vi "数据查询_报警信息.vi"() -> ()   [LabVIEW 2016, in "数据查询.lvlib"]
uses:
  <vilib>/Utility/miscctls.llb/LVPointTypeDef.ctl
  <vilib>/Utility/miscctls.llb/LVRowAndColumnUnsignedTypeDef.ctl
  <userlib>/_OpenG.lib/array/array.llb/Remove Duplicates from 1D Array (String)__ogtk.vi
  <userlib>/_OpenG.lib/array/array.llb/Sort 2D Array (String)__ogtk.vi
  <vilib>/addons/database/_DB Variant To Data/Database Variant To Data.xnode
panel:
  in  "列表框":i32(listbox)
  in  "页":i32 format="第%.0f页"
  in  "每页条数":i32=1000
  in  "向后按钮":bool
  in  "向前按钮":bool
  in  "导出":bool
  in  "查询":bool
  in  "结束日期":string="2050/01/01"
  in  "起始日期":string="2010/01/01"
  out "数据表":string[][](table)
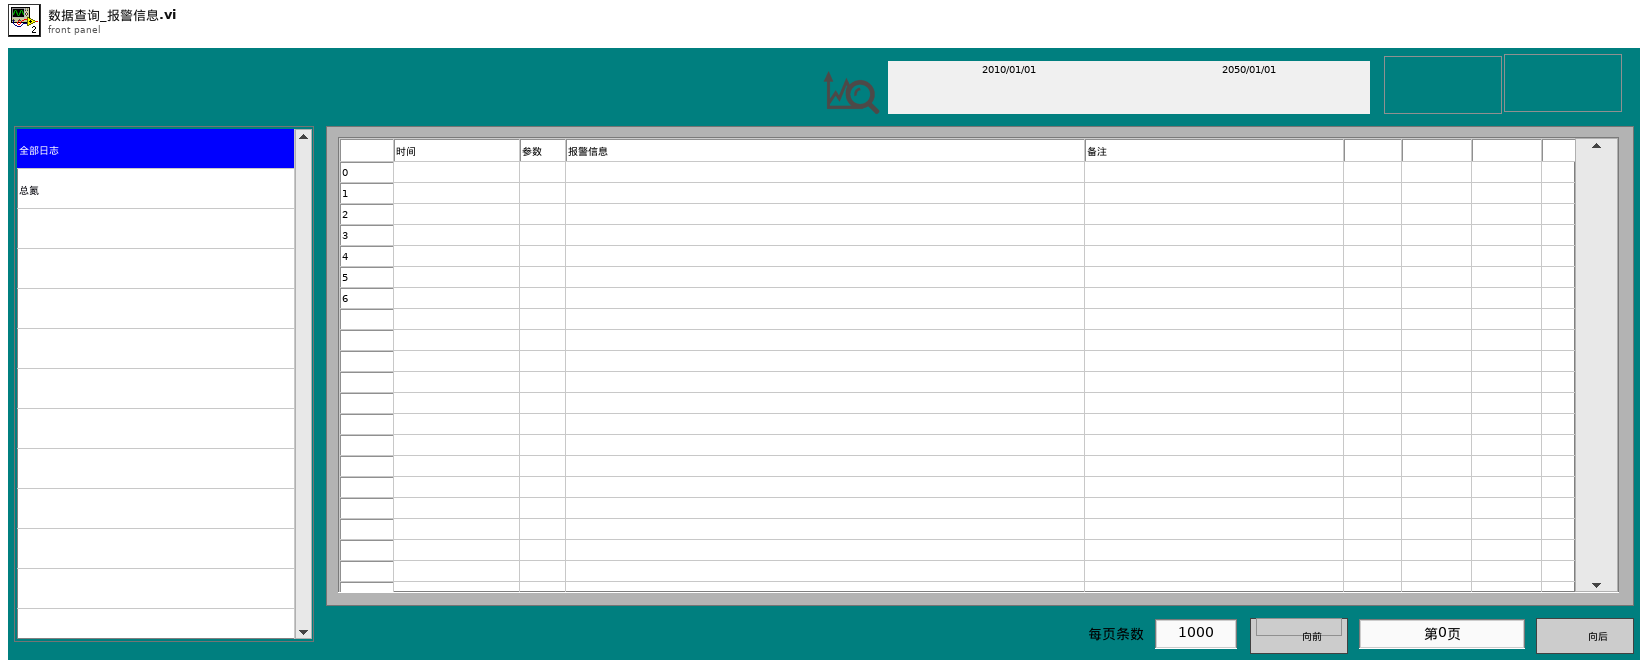
[diagram p1: front panel]
types:
  T1 = typedef "LVPointTypeDef.ctl" = cluster{"Horizontal":i16, "Vertical":i16}
  T2 = typedef "LVDateTimeRec.ctl" = cluster{"秒数的小数部分":dbl, "秒":i32, "分":i32, "时":i32, "日":i32, "月":i32, "年":i32, "天数（周）":i32, "天数（年）":i32, "DST":i32}
  T3 = enum8{"Enabled", "Disabled", "Disabled and Grayed Out"}
  T4 = typedef "LVRowAndColumnUnsignedTypeDef.ctl" = cluster{"Row":u32, "Column":u32}
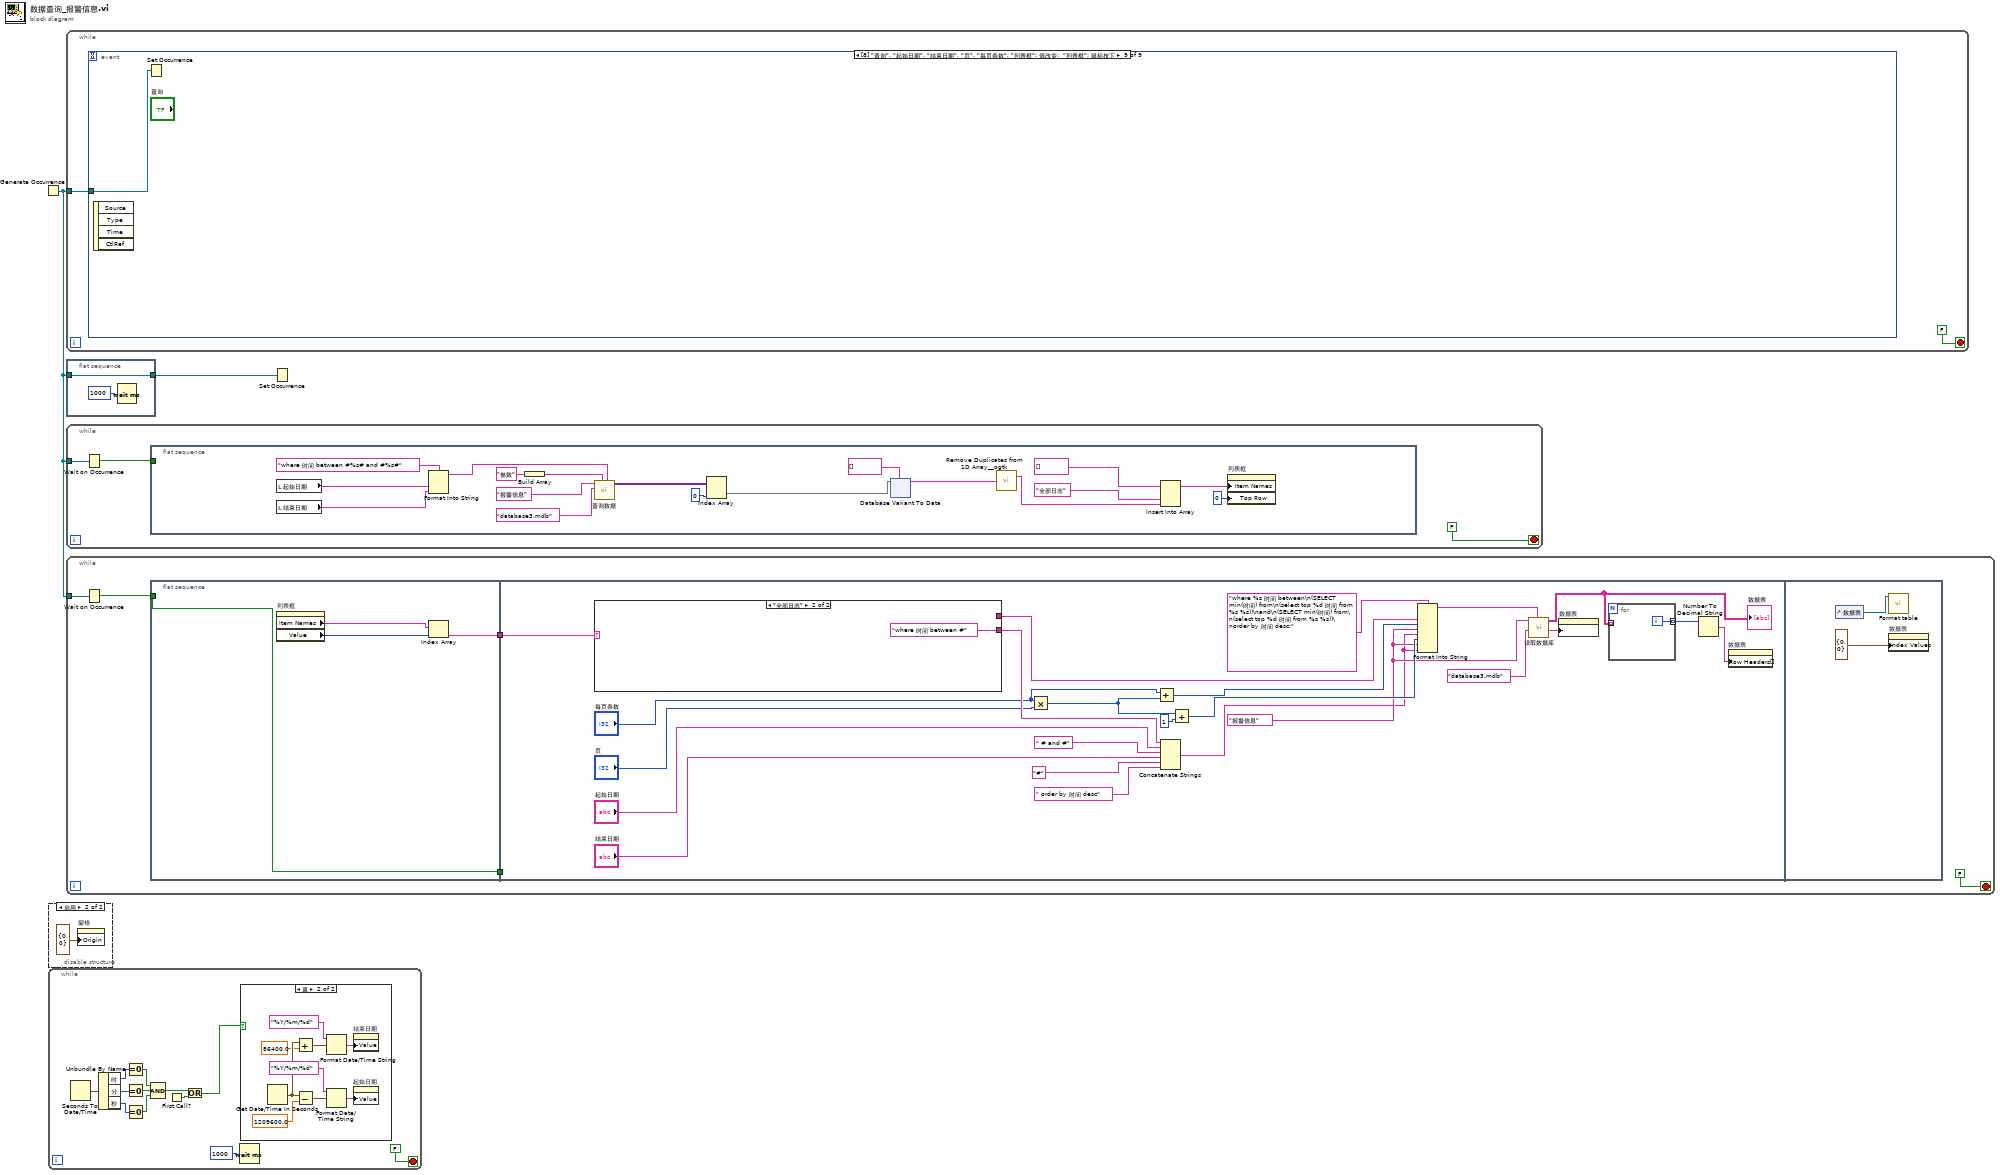
[diagram p0: block diagram]
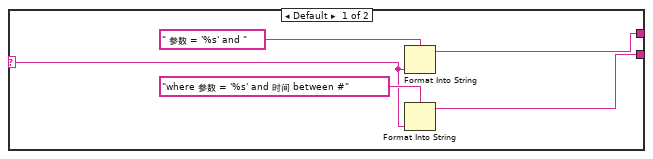
[diagram p2: hidden frame]
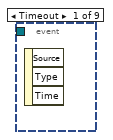
[diagram p4: hidden frame]
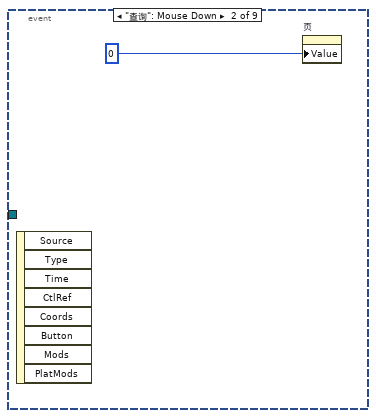
[diagram p5: hidden frame]
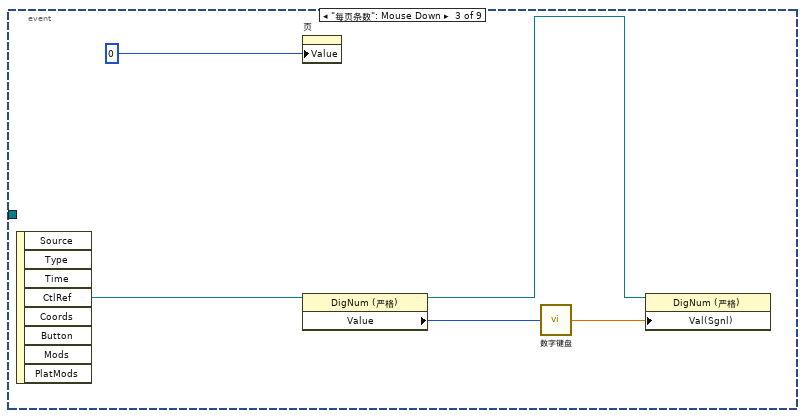
[diagram p6: hidden frame]
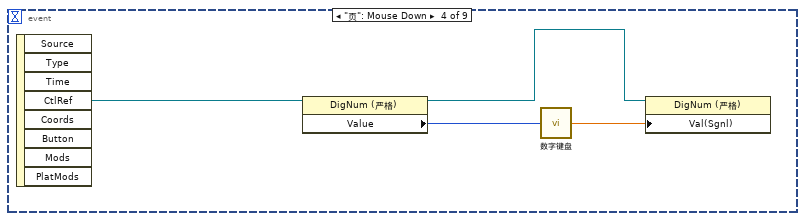
[diagram p7: hidden frame]
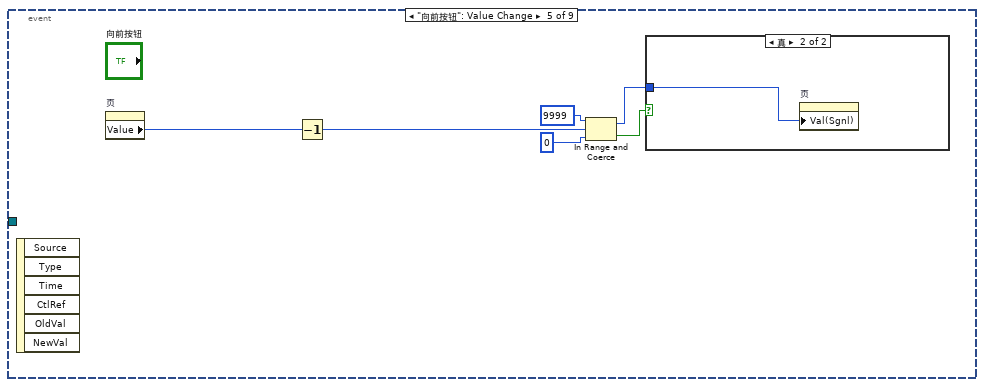
[diagram p8: hidden frame]
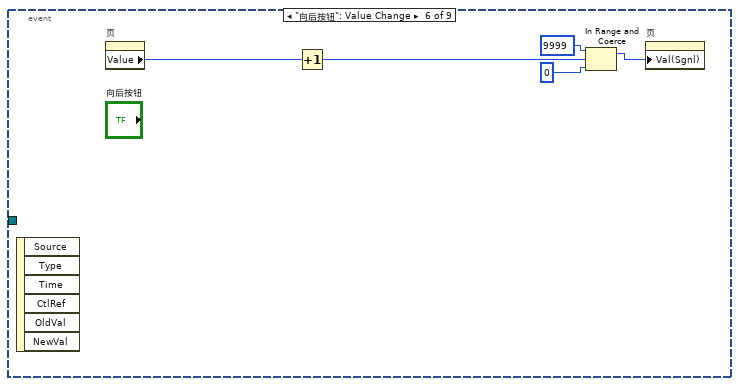
[diagram p10: hidden frame]
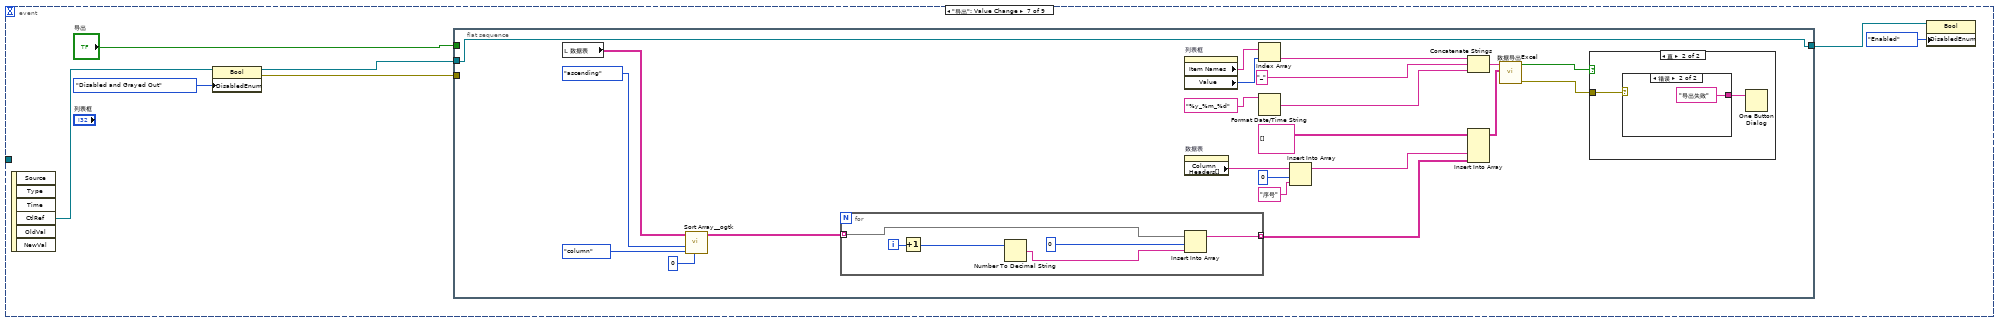
[diagram p11: hidden frame]
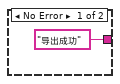
[diagram p13: hidden frame]
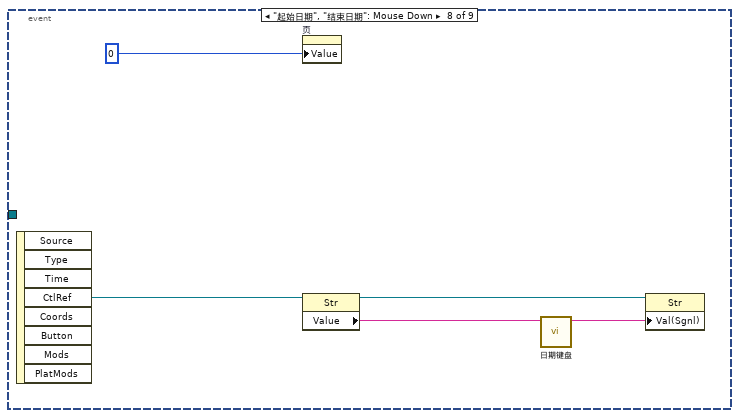
[diagram p14: hidden frame]
diagram:
  n1 = Generate Occurrence() -> (w1:refnum<k4>)
  n2 = disable-structure shown="启用" {
    frame Disabled {
    }
    frame Enabled {
      n3 = property on="窗格" class="Pane"("Origin"=T1 {"Horizontal"=0, "Vertical"=0} ("原点")) -> ()  [unwired: 2 in, 2 out]
    }
  }
  n4 = while {
    stop <- FALSE stop-if-true
    n5 = Seconds To Date/Time() -> (date time rec=w15:T2)  [unwired: 2 in]
    n6 = Unbundle By Name(w15) -> ("时"=w14:i32, "分"=w13:i32, "秒"=w12:i32)
    n7 = Equal To 0?(x=w14) -> (x = 0?=w11:bool)
    n8 = Equal To 0?(x=w13) -> (x = 0?=w10:bool)
    n9 = Equal To 0?(x=w12) -> (x = 0?=w9:bool)
    n10 = Compound Arithmetic op=AND ("复合运算")(w11, w10, w9) -> (w6:bool)
    n11 = First Call?() -> (First Call?: T/F=w5:bool)
    n12 = Or(x=w6, y=w5) -> (x .or. y?=w4:bool)
    n13 = Wait (ms)(milliseconds to wait=u32 1000 ("等待时间（毫秒）")) -> ()  [unwired: 1 out]
    n14 = case shown="真" w4 {
      frame False {
      }
      frame True {
        n15 = Get Date/Time In Seconds() -> (seconds since 1Jan1904=w20:timestamp)
        n16 = Add(x=w20, y=86400.0) -> (x+y=w18:timestamp)
        n17 = Subtract(x=w20, y=1209600.0) -> (x-y=w21:timestamp)
        n18 = Format Date/Time String(time format string (%c)="%Y/%m/%d" ("时间格式字符串(%c)"), seconds (now)=w18) -> (date/time string=w17:string)  [unwired: 1 in]
        n19 = Format Date/Time String(time format string (%c)="%Y/%m/%d" ("时间格式字符串(%c)"), seconds (now)=w21) -> (date/time string=w23:string)  [unwired: 1 in]
        n20 = property on="结束日期" class="Str"("Value"=w17) -> ()  [unwired: 2 in, 2 out]
        n21 = property on="起始日期" class="Str"("Value"=w23) -> ()  [unwired: 2 in, 2 out]
      }
    }
  }
  n22 = while {
    tunnel: w1 -> [w25]
    stop <- FALSE stop-if-true
    n23 = event shown="[8] \"查询\", \"起始日期\", \"结束日期\", \"页\", \"每页条数\", \"列表框\": 值改变;  \"列表框\": 鼠标按下" {
      selector: _ -> [_ _ _ _ _ _ _ _ _]
      dyn-events: _ -> [_ _ _ _ _ _ _ _ _]
      timeout: _ -> [_ _ _ _ _ _ _ _ _]
      tunnel: w25 -> [_ _ _ _ _ _ _ _ w93]
      event Timeout {
        n24 = event-data() -> ()  [unwired: 1 in, 3 out]
      }
      event "查询": Mouse Down {
        n25 = event-data() -> ()  [unwired: 1 in, 8 out]
        n26 = property on="页" class="DigNum (严格)"("Value"=0 ("页")) -> ()  [unwired: 2 in, 2 out]
      }
      event "每页条数": Mouse Down {
        n27 = event-data() -> ("CtlRef"=w29:refnum<vi>)  [unwired: 1 in, 7 out]
        n28 = property on="页" class="DigNum (严格)"("Value"=0 ("页")) -> ()  [unwired: 2 in, 2 out]
        n29 = property class="DigNum (严格)"(reference=w29) -> (reference out=w30:refnum<vi>, "Value"=w32:i32)  [unwired: 1 in, 1 out]
        n30 = call "数字键盘.vi"("OldNumber"=w32) -> ("NewNumber"=w31:sgl)
        n31 = property class="DigNum (严格)"(reference=w30, "Val(Sgnl)"=w31) -> ()  [unwired: 1 in, 2 out]
      }
      event "页": Mouse Down {
        n32 = event-data() -> ("CtlRef"=w33:refnum<vi>)  [unwired: 1 in, 7 out]
        n33 = property class="DigNum (严格)"(reference=w33) -> (reference out=w34:refnum<vi>, "Value"=w36:i32)  [unwired: 1 in, 1 out]
        n34 = call "数字键盘.vi"("OldNumber"=w36) -> ("NewNumber"=w35:sgl)
        n35 = property class="DigNum (严格)"(reference=w34, "Val(Sgnl)"=w35) -> ()  [unwired: 1 in, 2 out]
      }
      event "向前按钮": Value Change {
        n36 = event-data() -> ()  [unwired: 1 in, 6 out]
        n37 = property on="页" class="DigNum (严格)"() -> ("Value"=w42:i32)  [unwired: 2 in, 2 out]
        n38 = Decrement(x=w42) -> (x-1=w41:i32)
        n39 = In Range and Coerce(upper limit=9999 ("上限"), x=w41, lower limit=0 ("下限")) -> (coerced(x)=w38:i32, In Range?=w37:bool)
        n40 = case shown="真" w37 {
          tunnel: w38 -> [_ w43]
          frame False {
          }
          frame True {
            n41 = property on="页" class="DigNum (严格)"("Val(Sgnl)"=w43) -> ()  [unwired: 2 in, 2 out]
          }
        }
      }
      event "向后按钮": Value Change {
        n42 = event-data() -> ()  [unwired: 1 in, 6 out]
        n43 = property on="页" class="DigNum (严格)"() -> ("Value"=w48:i32)  [unwired: 2 in, 2 out]
        n44 = Increment(x=w48) -> (x+1=w47:i32)
        n45 = In Range and Coerce(upper limit=u32 9999 ("上限"), x=w47, lower limit=u32 0 ("下限")) -> (coerced(x)=w44:u32)  [unwired: 1 out]
        n46 = property on="页" class="DigNum (严格)"("Val(Sgnl)"=w44) -> ()  [unwired: 2 in, 2 out]
      }
      event "导出": Value Change {
        n47 = event-data() -> ("CtlRef"=w49:refnum<vi>)  [unwired: 1 in, 5 out]
        n48 = property class="Bool"(reference=w49, "DisabledEnum"=T3."Disabled and Grayed Out" ("禁用")) -> (reference out=w53:refnum<vi>, error out=w54:errorcluster)  [unwired: 1 in]
        n49 = flat-sequence {
          tunnel: w54 -> [_]
          tunnel: [w73] -> w52
          tunnel: w53 -> [w73]
          tunnel: "导出" -> [_]
          frame #0 {
            n50 = local read "数据表"() -> (w77:string[][])
            n51 = call-poly <userlib>:"Sort Array__ogtk.vi"("Column/Row to Sort By"=u32 0, "Sort By in"=enum16{"row", "column"}."column", "Order"=enum16{"ascending", "descending"}."ascending", "Array in"=w77) -> ("Sorted Array out"=w59:string[][])  [unwired: 4 in, 3 out]
            n52 = for {
              tunnel: w59 -> [w86] mode=indexing
              tunnel: [w85] -> w63 mode=indexing
              i -> [w87]
              n53 = Increment(x=w87) -> (x+1=w83:i32)
              n54 = Number To Decimal String(number=w83) -> (decimal integer string=w82:string)  [unwired: 1 in]
              n55 = Insert Into Array(array=w86, index=0 ("索引"), new element=w82) -> (w85:string[])
            }
            n56 = property on="列表框" class="LstBox (严格)"() -> ("Item Names"=w58:string[], "Value"=w57:i32)  [unwired: 2 in, 2 out]
            n57 = property on="数据表" class="Tbl (严格)"() -> ("Column Headers[]"=w66:string[])  [unwired: 2 in, 2 out]
            n58 = Index Array(array=w58, index=w57) -> (element=w56:string)
            n59 = Format Date/Time String(time format string (%c)="%y_%m_%d" ("时间格式字符串(%c)")) -> (date/time string=w70:string)  [unwired: 2 in]
            n60 = Insert Into Array(array=w66, index=0 ("索引"), new element="序号" ("新元素/子数组")) -> (w67:string[])
            n61 = Concatenate Strings(w56, "_" ("字符串"), w70) -> (w68:string)
            n62 = Insert Into Array(array=string[][] [], new element #1=w67, new element #2=w63) -> (w62:string[][])  [unwired: 2 in]
            n63 = call "数据导出Excel.vi"("text data"=w62, "default name"=w68) -> ("error out"=w61:errorcluster, "布尔"=w60:bool)  [unwired: 8 in]
            n64 = case shown="真" w60 {
              tunnel: w61 -> [_ w79]
              frame False {
              }
              frame True {
                n65 = case shown="错误" w79 {
                  tunnel: ["导出成功" ("消息") "导出失败" ("消息")] -> w78
                  frame No Error {
                  }
                  frame Error {
                  }
                }
                n66 = One Button Dialog(message=w78) -> ()  [unwired: 1 in, 1 out]
              }
            }
          }
        }
        n67 = property class="Bool"(reference=w52, "DisabledEnum"=T3."Enabled" ("禁用")) -> ()  [unwired: 1 in, 2 out]
      }
      event "起始日期", "结束日期": Mouse Down {
        n68 = event-data() -> ("CtlRef"=w92:refnum<vi>)  [unwired: 1 in, 7 out]
        n69 = property on="页" class="DigNum (严格)"("Value"=0 ("页")) -> ()  [unwired: 2 in, 2 out]
        n70 = property class="Str"(reference=w92) -> (reference out=w90:refnum<vi>, "Value"=w91:string)  [unwired: 1 in, 1 out]
        n71 = call "日期键盘.vi"("原值"=w91) -> ("x+y"=w89:string)  [unwired: 10 in]
        n72 = property class="Str"(reference=w90, "Val(Sgnl)"=w89) -> ()  [unwired: 1 in, 2 out]
      }
      event "查询", "起始日期", "结束日期", "页", "每页条数", "列表框": Value Change; "列表框": Mouse Down {
        n73 = event-data() -> ()  [unwired: 1 in, 4 out]
        n74 = Set Occurrence(w93) -> ()
      }
    }
  }
  n75 = flat-sequence {
    tunnel: w1 -> [w95]
    tunnel: [w95] -> w2
    frame #0 {
      n76 = Wait (ms)(milliseconds to wait=u32 1000 ("等待时间（毫秒）")) -> ()  [unwired: 1 out]
    }
  }
  n77 = while {
    tunnel: w1 -> [w96]
    stop <- FALSE stop-if-true
    n78 = Wait on Occurrence(2:w96) -> (0:w97:bool)  [unwired: 2 in]
    n79 = flat-sequence {
      tunnel: w97 -> [_]
      frame #0 {
        n80 = local read "起始日期"() -> (w102:string)
        n81 = local read "结束日期"() -> (w101:string)
        n82 = Format Into String(format string="where 时间 between #%s# and #%s#" ("格式字符串"), w102, w101) -> (resulting string=w103:string)  [unwired: 2 in, 1 out]
        n83 = Build Array("参数") -> (w111:string[])
        n84 = call "查询数据.vi"("condition"=w103, "columns"=w111, "database"="database3.mdb", "table"="报警信息") -> ("data"=w110:variant[][])  [unwired: 6 in, 1 out]
        n85 = Index Array(array=w110, index (col)=0 ("禁用的索引 (列)")) -> (element=w109:variant[])  [unwired: 1 in]
        n86 = xnode "Database Variant To Data"("database variant"=w109, "type"=string[] []) -> ("data"=w106:string[])  [unwired: 1 in, 1 out]
        n87 = call-poly <userlib>:"Remove Duplicates from 1D Array__ogtk.vi"("Input Array"=w106) -> ("Output Array"=w105:string[])  [unwired: 1 out]
        n88 = Insert Into Array(array=string[] [], new element #1="全部日志" ("新元素/子数组"), new element #2=w105) -> (w100:string[])  [unwired: 1 in]
        n89 = property on="列表框" class="LstBox (严格)"("Item Names"=w100, "Top Row"=0 ("顶行")) -> ()  [unwired: 2 in, 2 out]
      }
    }
  }
  n90 = while {
    tunnel: w1 -> [w158]
    stop <- FALSE stop-if-true
    n91 = Wait on Occurrence(2:w158) -> (0:w157:bool)  [unwired: 2 in]
    n92 = flat-sequence {
      tunnel: w157 -> [w163]
      tunnel: [w163] -> w156
      tunnel: [w160] -> w155
      tunnel: w156 -> [_]
      tunnel: w155 -> [w164]
      frame #0 {
        n93 = property on="列表框" class="LstBox (严格)"() -> ("Item Names"=w162:string[], "Value"=w161:i32)  [unwired: 2 in, 2 out]
        n94 = Index Array(array=w162, index=w161) -> (element=w160:string)
      }
      frame #1 {
        w168 = "报警信息" ("组合框")
        n95 = case shown="\"全部日志\"" w164 {
          selector: w164 -> [w188 _]
          tunnel: [w191 "where 时间 between #" ("condition")] -> w176
          tunnel: [w187 _] -> w165
          frame Default {
            n96 = Format Into String(format string=" 参数 = '%s' and " ("condition"), w188) -> (resulting string=w187:string)  [unwired: 2 in, 1 out]
            n97 = Format Into String(format string="where 参数 = '%s' and 时间 between #" ("condition"), w188) -> (resulting string=w191:string)  [unwired: 2 in, 1 out]
          }
          frame "全部日志" {
          }
        }
        n98 = Multiply(x="每页条数", y="页") -> (x*y=w174:i32)
        n99 = Add(x="每页条数", y=w174) -> (x+y=w172:i32)
        n100 = Concatenate Strings(w176, "起始日期", " # and #" ("condition"), "结束日期", "#" ("condition"), " order by 时间 desc" ("字符串")) -> (w167:string)
        n101 = Add(x=w174, y=u32 1) -> (x+y=w171:u32)
        n102 = Format Into String(format string="where %s 时间 between\n(SELECT min(时间) from\n(select top %d 时间 from %s %s))\nand\n(SELECT min(时间) from\n(select top %d 时间 from %s %s))\norder by 时间 desc;" ("格式字符串"), w165, w172, w168, w167, w171, w168, w167) -> (resulting string=w166:string)  [unwired: 2 in, 1 out]
        n103 = call "读取数据库.vi"("condition"=w166, "database"="database3.mdb", "组合框"=w168) -> ("columns"=w182:string[], "表格"=w180:string[][])  [unwired: 5 in, 2 out]
        "数据表" <- w180
        n104 = property on="数据表" class="Tbl (严格)"("Column Headers[]"=w182) -> ()  [unwired: 2 in, 2 out]
        n105 = for {
          tunnel: w180 -> [_] mode=indexing
          tunnel: [w193] -> w179 mode=indexing
          i -> [w193]
        }
        n106 = Number To Decimal String(number=w179) -> (decimal integer string=w178:string[])  [unwired: 1 in]
        n107 = property on="数据表" class="Tbl (严格)"("Row Headers[]"=w178) -> ()  [unwired: 2 in, 2 out]
      }
      frame #2 {
        n108 = control-ref of="数据表"() -> (w194:refnum<vi>)
        n109 = call "Format table.vi"("Table输入"=w194) -> ()  [unwired: 11 in]
        n110 = property on="数据表" class="Tbl (严格)"("Index Values"=T4 {"Row"=0, "Column"=0} ("索引值")) -> ()  [unwired: 2 in, 2 out]
      }
    }
  }
  n111 = Set Occurrence(w2) -> ()
